vi "WriteAttrib.vi"(11 "Data In":T1={"DAQ Config Data"={"Vertical"={"Coupling"=1, "Offset (V)"=-0.5, "Range (V)"=2.0, "Impedance"=50.0}, "Horizontal"={"Offset Time"=0.0, "Sample Time (S)"=22.0, "Sample Points"=1000}, "Trigger\n"={"Lower Level (V)"=-0.02, "Trigger Slope"=1, "Trigger Source"=10}, "Acquisition"={"Trigger Mode"=1, "Initiate Continuously"=0, "Acquire Type"=0, "Acquire Count"=1}, "Channel"=0, "Instrument Handle"=0, "Error"={"status"=FALSE, "code"=0, "source"=""}, "State"=1}, "Acquisition"={"Current"={"Acquiring Now?"=FALSE, "Waveforms Acquired"=0.0, "Start of Acquisition"=timestamp(0 s since 1904-01-01), "Acquisition Name"=""}, "Stop Condition"={"Quota"=3000.0, "Duration (S)"=22, "Stop Condition"=FALSE}, "Config Needed"=FALSE}, "Measurement"={"Waveform"={"t0"=timestamp(0 s since 1904-01-01), "dt"=1.0, "Y"=[]}, "Peak Heights"=[], "Acquisition Time"=timestamp(0 s since 1904-01-01), "File Path"=path "C:/Users/lab-341/Desktop/Reed/Oscilloscope VI/pulses.tdms", "TDMS File Handle"=refnum}, "UI References"={"Acquire"=refnum, "Configure DAQ"=refnum, "Measurement (Ch1)"=refnum, "Update Needed?"=FALSE, "New Run"=refnum, "Signal"=refnum}, "Run Info"={"Active Run?"=FALSE, "Run Notes"="Enter in notes explaining the purpose of the run and any unusual steps taken in the process. This should make it clear why the data was taken. e.g. \"Measuring LXe scintillation light with Teflon\" or \"Measuring dark pulses to determine SPE gain.\" Concise is good but precise is better.", "User Name"="", "Campaign ID#"="", "Run Name"="", "Start Time"=timestamp(0 s since 1904-01-01), "End Time"=timestamp(0 s since 1904-01-01)}, "System Status"={"Bias Voltage"=0.0, "SiPM Temperature"=[], "Slow Control User"="", "LXe"=0.0}, "Acquisition Info"={"Trigger Mode"=FALSE, "Acquisition Mode"=FALSE, "Bias Voltage (V)"=0.0, "Preamplifier"=0, "Shaping Amplifier"=0, "Acquisition Notes"="", "1"=FALSE, "2"=FALSE}} {"Acquisition Info"."Shaping Amplifier" items=["CR-200-100ns", "CR-200-1us"]; "Acquisition Info"."Preamplifier" items=["CR-Z-113-1k", "CR-Z-113-5k", "CR-Z-SiPM"]; "DAQ Config Data"."State" items=["Enable"=1, "Disable"=0]; "DAQ Config Data"."Channel" items=["Input Channel 1", "Input Channel 2", "Input Channel 3", "Input Channel 4"]; "DAQ Config Data"."Acquisition"."Acquire Type" items=["Normal"=0, "Average"=1, "Envelope"=2, "Peak Detect"=3, "High Resolution"=4, "Fast"=5, "Equivalent Time"=16]; "DAQ Config Data"."Acquisition"."Initiate Continuously" items=["Continuously"=1, "Single Capture"=0]; "DAQ Config Data"."Acquisition"."Trigger Mode" items=["Auto", "Normal"]; "DAQ Config Data"."Trigger"."Trigger Source" items=["TTL0", "TTL1", "TTL2", "TTL3", "TTL4", "TTL5", "TTL6", "TTL7", "ECL0", "ECL1", "Input Channel 1", "Input Channel 2", "Input Channel 3", "Input Channel 4", "External Trigger Source", "STAR", "Manual Trigger", "Pattern"]; "DAQ Config Data"."Trigger"."Trigger Slope" items=["Rising Edge", "Falling Edge"]; "DAQ Config Data"."Horizontal"."Sample Time (S)" items=["0.5"=0.5, "0.4"=0.4, "0.25"=0.25, "0.2"=0.2, "0.1"=0.1, "0.05"=0.05, "0.04"=0.04, "0.025"=0.025, "0.02"=0.02, "0.01"=0.01, "0.005"=0.005, "0.004"=0.004, "0.0025"=0.0025, "0.002"=0.002, "0.001"=0.001, "5E-4"=0.0005, "4E-4"=0.0004, "2.5E-4"=0.00025, "2E-4"=0.0002, "1E-4"=0.0001, "5E-5"=5e-05, "4E-5"=4e-05, "2E-5"=2e-05, "5E-6"=5e-06, "1E-6"=1e-06, "5E-7"=5e-07, "1E-7"=1e-07, "5E-8"=5e-08, "1E-8"=1e-08]; "DAQ Config Data"."Vertical"."Impedance" items=["50 Ohm"=50.0, "1 MOhm"=1000000.0]; "DAQ Config Data"."Vertical"."Range (V)" items=["10"=10.0, "5"=5.0, "2"=2.0, "1"=1.0, "0.4"=0.4, "0.2"=0.2, "0.08"=0.08, "0.04"=0.04, "0.02"=0.02, "0.01"=0.01]; "DAQ Config Data"."Vertical"."Coupling" items=["AC", "DC"]}) -> ()   [LabVIEW 2012]
uses:
  TypeDefs/DataTypes/Data.ctl
  TypeDefs/DataTypes/DAQConfig.ctl
  TypeDefs/DataTypes/Acquisition.ctl
  TypeDefs/DataTypes/Current.ctl
  TypeDefs/DataTypes/StopCondition.ctl
  TypeDefs/DataTypes/Measurement.ctl
  TypeDefs/DataTypes/UIReferences.ctl
  TypeDefs/DataTypes/RunInfo.ctl
  TypeDefs/DataTypes/SystemStatus.ctl
  <vilib>/addons/h5labview2/file/H5Fmode.ctl
  <vilib>/addons/h5labview2/base/lib_path.vi
  <vilib>/addons/h5labview2/base/H5Equery.vi
  <vilib>/addons/h5labview2/attrib/H5Awrite.llb/H5Awrite.xnode
  <vilib>/addons/h5labview2/file/H5F.lvlib
  <vilib>/addons/h5labview2/group/H5G.lvlib
panel:
  # "Open the H5File created by NewH5File.vi\nThen create a group in the file for acquisition named Acquisition_{integer rep of start time in UTC}\nThen write all acquisition-specific attributes"
  # "Shaper Gain"
  # "Self"
  # "Fast"
  # "Solicited"
  # "Standard"
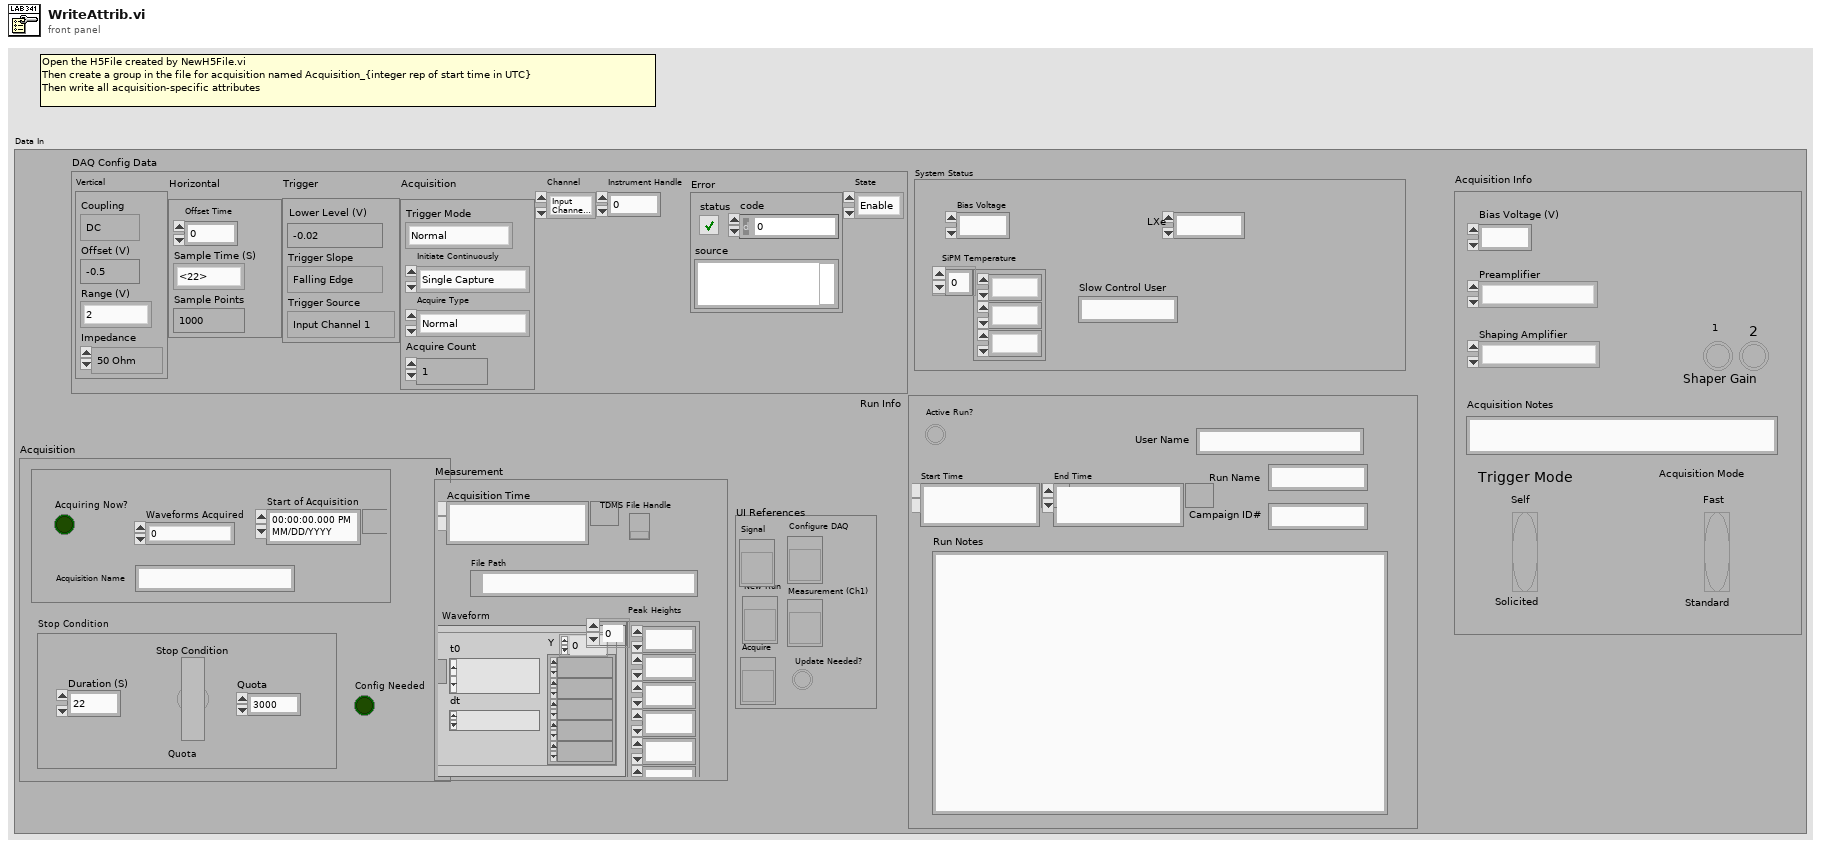
[diagram p1: front panel]
types:
  T1 = typedef "Data.ctl" = cluster{"DAQ Config Data":T2, "Acquisition":T3, "Measurement":T6, "UI References":T7, "Run Info":T8, "System Status":T9, "Acquisition Info":cluster{"Trigger Mode":bool, "Acquisition Mode":bool, "Bias Voltage (V)":dbl, "Preamplifier":u16, "Shaping Amplifier":u16, "Acquisition Notes":string, "1":bool, "2":bool}}
  T2 = typedef "DAQConfig.ctl" = cluster{"Vertical":cluster{"Coupling":i32, "Offset (V)":dbl, "Range (V)":dbl, "Impedance":dbl}, "Horizontal":cluster{"Offset Time":dbl, "Sample Time (S)":dbl, "Sample Points":u32}, "Trigger\n":cluster{"Lower Level (V)":dbl, "Trigger Slope":i32, "Trigger Source":i32}, "Acquisition":cluster{"Trigger Mode":i32, "Initiate Continuously":i32, "Acquire Type":i32, "Acquire Count":i32}, "Channel":i32, "Instrument Handle":i32, "Error":errorcluster, "State":i32}
  T3 = typedef "Acquisition.ctl" = cluster{"Current":T4, "Stop Condition":T5, "Config Needed":bool}
  T4 = typedef "Current.ctl" = cluster{"Acquiring Now?":bool, "Waveforms Acquired":dbl, "Start of Acquisition":timestamp, "Acquisition Name":string}
  T5 = typedef "StopCondition.ctl" = cluster{"Quota":dbl, "Duration (S)":u16, "Stop Condition":bool}
  T6 = typedef "Measurement.ctl" = cluster{"Waveform":waveform(dbl), "Peak Heights":dbl[], "Acquisition Time":timestamp, "File Path":path, "TDMS File Handle":refnum<k34>}
  T7 = typedef "UIReferences.ctl" = cluster{"Acquire":refnum<vi>, "Configure DAQ":refnum<vi>, "Measurement (Ch1)":refnum<vi>, "Update Needed?":bool, "New Run":refnum<vi>, "Signal":refnum<vi>}
  T8 = typedef "RunInfo.ctl" = cluster{"Active Run?":bool, "Run Notes":string, "User Name":string, "Campaign ID#":string, "Run Name":string, "Start Time":timestamp, "End Time":timestamp}
  T9 = typedef "SystemStatus.ctl" = cluster{"Bias Voltage":dbl, "SiPM Temperature":dbl[], "Slow Control User":string, "LXe":dbl}
  T10 = typedef "H5F.lvlib/H5Fmode.ctl" = enum16{"read-only", "read-write", "overwrite", "create new", "open or create"}
  T11 = typedef "hid_t.ctl" = i64
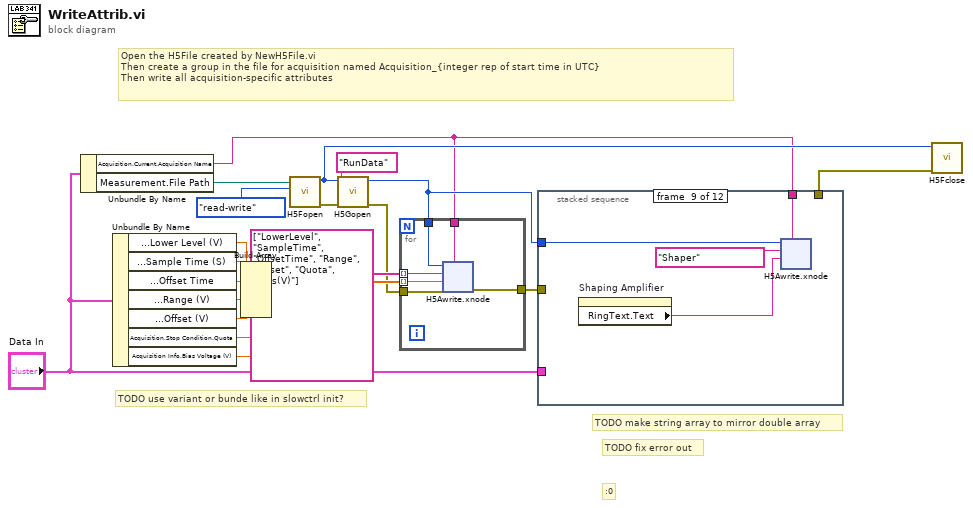
[diagram p0: block diagram]
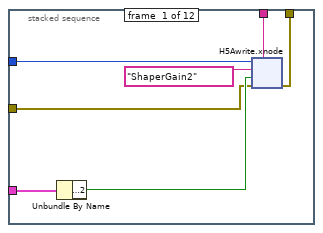
[diagram p2: hidden frame]
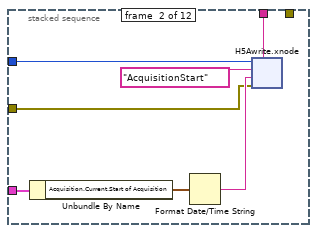
[diagram p3: hidden frame]
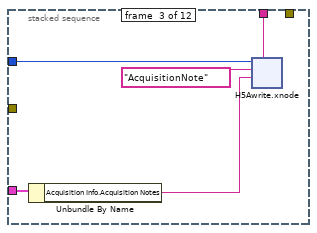
[diagram p4: hidden frame]
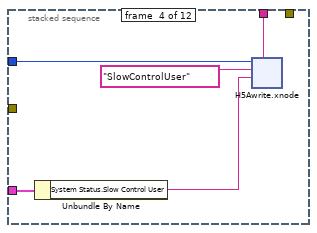
[diagram p5: hidden frame]
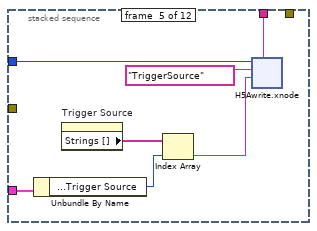
[diagram p6: hidden frame]
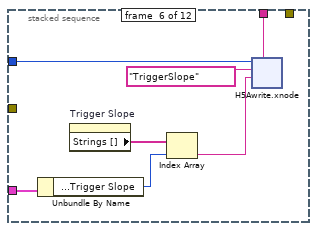
[diagram p7: hidden frame]
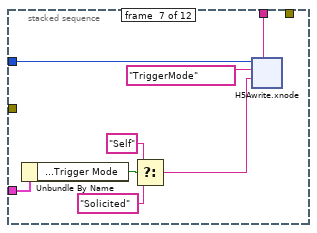
[diagram p8: hidden frame]
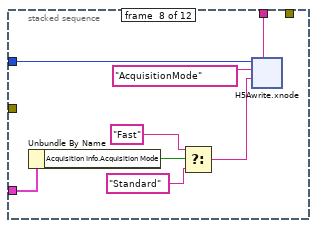
[diagram p9: hidden frame]
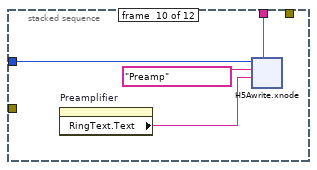
[diagram p10: hidden frame]
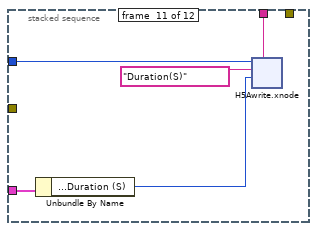
[diagram p11: hidden frame]
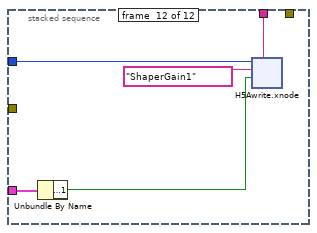
[diagram p12: hidden frame]
diagram:
  # "TODO fix error out"
  # "TODO use variant or bunde like in slowctrl init?"
  # "TODO make string array to mirror double array"
  # ":0"
  # "Open the H5File created by NewH5File.vi\nThen create a group in the file for acquisition named Acquisition_{integer rep of start time in UTC}\nThen write all acquisition-specific attributes"
  n1 = Unbundle By Name("Data In") -> ("Acquisition.Current.Acquisition Name"=w1:string, "Measurement.File Path"=w20:path)
  n2 = Unbundle By Name("Data In") -> ("DAQ Config Data.Trigger.Lower Level (V)"=w17:dbl, "DAQ Config Data.Horizontal.Sample Time (S)"=w16:dbl, "DAQ Config Data.Horizontal.Offset Time"=w15:dbl, "DAQ Config Data.Vertical.Range (V)"=w14:dbl, "DAQ Config Data.Vertical.Offset (V)"=w13:dbl, "Acquisition.Stop Condition.Quota"=w12:dbl, "Acquisition Info.Bias Voltage (V)"=w4:dbl)
  n3 = Build Array(w17, w16, w15, w14, w13, w12, w4) -> (w11:dbl[])
  n4 = call <vilib>:"H5Fopen.vi"("mode (read-only)"=H5Fmode."read-write", "path"=w20) -> ("error out"=w10:errorcluster, "ref out"=w9:T11)  [unwired: 8 in]
  n5 = call <vilib>:"H5Gopen.vi"("error in (no error)"=w10, "name"="RunData", "ref in"=w9) -> ("error out"=w8:errorcluster, "group out"=w5:T11)  [unwired: 7 in]
  n6 = for {
    tunnel: string[] ["LowerLevel", "SampleTime", "OffsetTime", "Range", "Offset", "Quota", "Bias(V)"] ("property names") -> [w26] mode=indexing
    tunnel: w11 -> [w25] mode=indexing
    tunnel: w5 -> [w24]
    tunnel: w8 -> [w23]
    tunnel: [w22] -> w7
    tunnel: w1 -> [w21]
    n7 = xnode "H5Awrite.xnode"("object name"=w21, "error in (no error)"=w23, "data"=w25, "attrib name"=w26, "ref in"=w24) -> ("error out"=w22:errorcluster)  [unwired: 2 in, 2 out]
  }
  n8 = stacked-sequence {
    tunnel: "Data In" -> [w50 w77 w100 w125 w150 w176 w203 w230 _ _ w300 w324]
    tunnel: w5 -> [w52 w78 w102 w126 w152 w178 w205 w232 w255 w278 w302 w326]
    tunnel: w7 -> [w46 w72 _ _ _ _ _ _ _ _ _ _]
    tunnel: [w47 _ _ _ _ _ _ _ _ _ _ _] -> w6
    tunnel: w1 -> [w48 w73 w98 w122 w146 w172 w198 w225 w253 w275 w298 w322]
    frame #0 {
      n9 = Unbundle By Name(w50) -> ("Acquisition Info.2"=w49:bool)
      n10 = xnode "H5Awrite.xnode"("object name"=w48, "error in (no error)"=w46, "data"=w49, "attrib name"="ShaperGain2", "ref in"=w52) -> ("error out"=w47:errorcluster)  [unwired: 2 in, 2 out]
    }
    frame #1 {
      n11 = Unbundle By Name(w77) -> ("Acquisition.Current.Start of Acquisition"=w75:timestamp)
      n12 = Format Date/Time String(seconds (now)=w75) -> (date/time string=w74:string)  [unwired: 2 in]
      n13 = xnode "H5Awrite.xnode"("object name"=w73, "error in (no error)"=w72, "data"=w74, "attrib name"="AcquisitionStart", "ref in"=w78) -> ()  [unwired: 2 in, 3 out]
    }
    frame #2 {
      n14 = Unbundle By Name(w100) -> ("Acquisition Info.Acquisition Notes"=w99:string)
      n15 = xnode "H5Awrite.xnode"("object name"=w98, "data"=w99, "attrib name"="AcquisitionNote", "ref in"=w102) -> ()  [unwired: 3 in, 3 out]
    }
    frame #3 {
      n16 = Unbundle By Name(w125) -> ("System Status.Slow Control User"=w123:string)
      n17 = xnode "H5Awrite.xnode"("object name"=w122, "data"=w123, "attrib name"="SlowControlUser", "ref in"=w126) -> ()  [unwired: 3 in, 3 out]
    }
    frame #4 {
      n18 = Unbundle By Name(w150) -> ("DAQ Config Data.Trigger.Trigger Source"=w149:i32)
      n19 = property on="Trigger Source" class="Ring (strict)"() -> ("Strings []"=w148:string[])  [unwired: 2 in, 2 out]
      n20 = Index Array(array=w148, index=w149) -> (element=w147:string)
      n21 = xnode "H5Awrite.xnode"("object name"=w146, "data"=w147, "attrib name"="TriggerSource", "ref in"=w152) -> ()  [unwired: 3 in, 3 out]
    }
    frame #5 {
      n22 = Unbundle By Name(w176) -> ("DAQ Config Data.Trigger.Trigger Slope"=w175:i32)
      n23 = property on="Trigger Slope" class="Ring (strict)"() -> ("Strings []"=w174:string[])  [unwired: 2 in, 2 out]
      n24 = Index Array(array=w174, index=w175) -> (element=w173:string)
      n25 = xnode "H5Awrite.xnode"("object name"=w172, "data"=w173, "attrib name"="TriggerSlope", "ref in"=w178) -> ()  [unwired: 3 in, 3 out]
    }
    frame #6 {
      n26 = Unbundle By Name(w203) -> ("Acquisition Info.Trigger Mode"=w202:bool)
      n27 = Select(t="Self", s=w202, f="Solicited") -> (s? t:f=w199:string)
      n28 = xnode "H5Awrite.xnode"("object name"=w198, "data"=w199, "attrib name"="TriggerMode", "ref in"=w205) -> ()  [unwired: 3 in, 3 out]
    }
    frame #7 {
      n29 = Unbundle By Name(w230) -> ("Acquisition Info.Acquisition Mode"=w227:bool)
      n30 = Select(t="Fast", s=w227, f="Standard") -> (s? t:f=w226:string)
      n31 = xnode "H5Awrite.xnode"("object name"=w225, "data"=w226, "attrib name"="AcquisitionMode", "ref in"=w232) -> ()  [unwired: 3 in, 3 out]
    }
    frame #8 {
      n32 = property on="Shaping Amplifier" class="Ring (strict)"() -> ("RingText.Text"=w252:string)  [unwired: 2 in, 2 out]
      n33 = xnode "H5Awrite.xnode"("object name"=w253, "data"=w252, "attrib name"="Shaper", "ref in"=w255) -> ()  [unwired: 3 in, 3 out]
    }
    frame #9 {
      n34 = property on="Preamplifier" class="Ring (strict)"() -> ("RingText.Text"=w276:string)  [unwired: 2 in, 2 out]
      n35 = xnode "H5Awrite.xnode"("object name"=w275, "data"=w276, "attrib name"="Preamp", "ref in"=w278) -> ()  [unwired: 3 in, 3 out]
    }
    frame #10 {
      n36 = Unbundle By Name(w300) -> ("Acquisition.Stop Condition.Duration (S)"=w299:u16)
      n37 = xnode "H5Awrite.xnode"("object name"=w298, "data"=w299, "attrib name"="Duration(S)", "ref in"=w302) -> ()  [unwired: 3 in, 3 out]
    }
    frame #11 {
      n38 = Unbundle By Name(w324) -> ("Acquisition Info.1"=w323:bool)
      n39 = xnode "H5Awrite.xnode"("object name"=w322, "data"=w323, "attrib name"="ShaperGain1", "ref in"=w326) -> ()  [unwired: 3 in, 3 out]
    }
  }
  n40 = call <vilib>:"H5Fclose.vi"("error in (no error)"=w6, "ref"=w9) -> ()  [unwired: 9 in, 1 out]
